vi "Teleop.vi"(10 "Match Info":T1={"Autonomous Elapsed Seconds"=0.0, "TeleOp Elapsed Seconds"=0.0, "Disabled Elapsed Seconds"=0.0, "Visited Autonomous"=FALSE, "Visited TeleOp"=FALSE, "Visited Disabled"=FALSE, "Autonomous Settings"={"Autonomous Style"=enum."Independent", "VI Refnum"=refnum}}, 11 "Call Context":T2) -> ()   [LabVIEW 2013]
doc: "This VI is called for each TeleOp packet received from the DS where the robot is not disabled. It is often used to read from the joysticks and update I/O or to update setpoints for timed control loops. It should complete and return within 20 milliseconds or it may miss DS packets."
uses:
  <vilib>/Rock Robotics/WPI/DriverStation/WPI_DriverStationDerivedRobotMode.ctl
  <vilib>/Rock Robotics/WPI/DriverStation/WPI_DriverStationMatch Info.ctl
  <vilib>/Rock Robotics/WPI/DriverStation/DriverStationLCD/WPI_DriverStationLCDLCDLine.ctl
  Begin/Robot Global Data.vi
  Begin/Global Refnums.vi
  Begin/Global Variables.vi
  <vilib>/Rock Robotics/WPI/Joystick/WPI_JoystickGetSetRefNum.vi
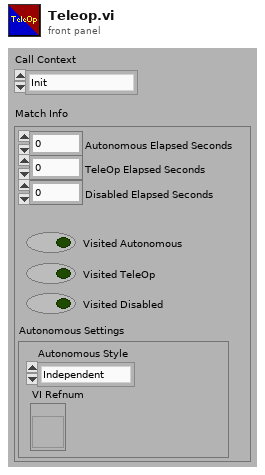
[diagram p1: front panel]
types:
  T1 = typedef "WPI_DriverStationMatch Info.ctl" = cluster{"Autonomous Elapsed Seconds":dbl, "TeleOp Elapsed Seconds":dbl, "Disabled Elapsed Seconds":dbl, "Visited Autonomous":bool, "Visited TeleOp":bool, "Visited Disabled":bool, "Autonomous Settings":cluster{"Autonomous Style":enum16{"Iterative", "Independent"}, "VI Refnum":refnum<vi>}}
  T2 = typedef "WPI_DriverStationDerivedRobotMode.ctl" = enum16{"Init", "Execute", "Stop"}
  T3 = typedef "WPI_DriverStationLCDLCDLine.ctl" = enum16{"Main - Line 1", "User - Line 2", "User - Line 3", "User - Line 4", "User - Line 5", "User - Line 6"}
  T4 = typedef "WPI_GyroDevRef.ctl" = cluster{"DevStatus":errorcluster, "Analog Module":T5, "Analog Channel":T6, "Offset":dbl, "Gain (VoltsPerDegree/Second)":dbl}
  T5 = typedef "FPGA_TypedefAnalogModule.ctl" = enum16{"Analog Module 1", "Analog Module 2"}
  T6 = typedef "FPGA_AIChannel.ctl" = enum8{"AI 1", "AI 2", "AI 3", "AI 4", "AI 5", "AI 6", "AI 7", "AI 8", "Invalid"}
  T7 = typedef "WPI_JoystickDevRef.ctl" = cluster{"Device":T8}
  T8 = typedef "WPI_JoystickDeviceEnum.ctl" = enum16{"USB 1", "USB 2", "USB 3", "USB 4", "Kinect 1", "Kinect 2"}
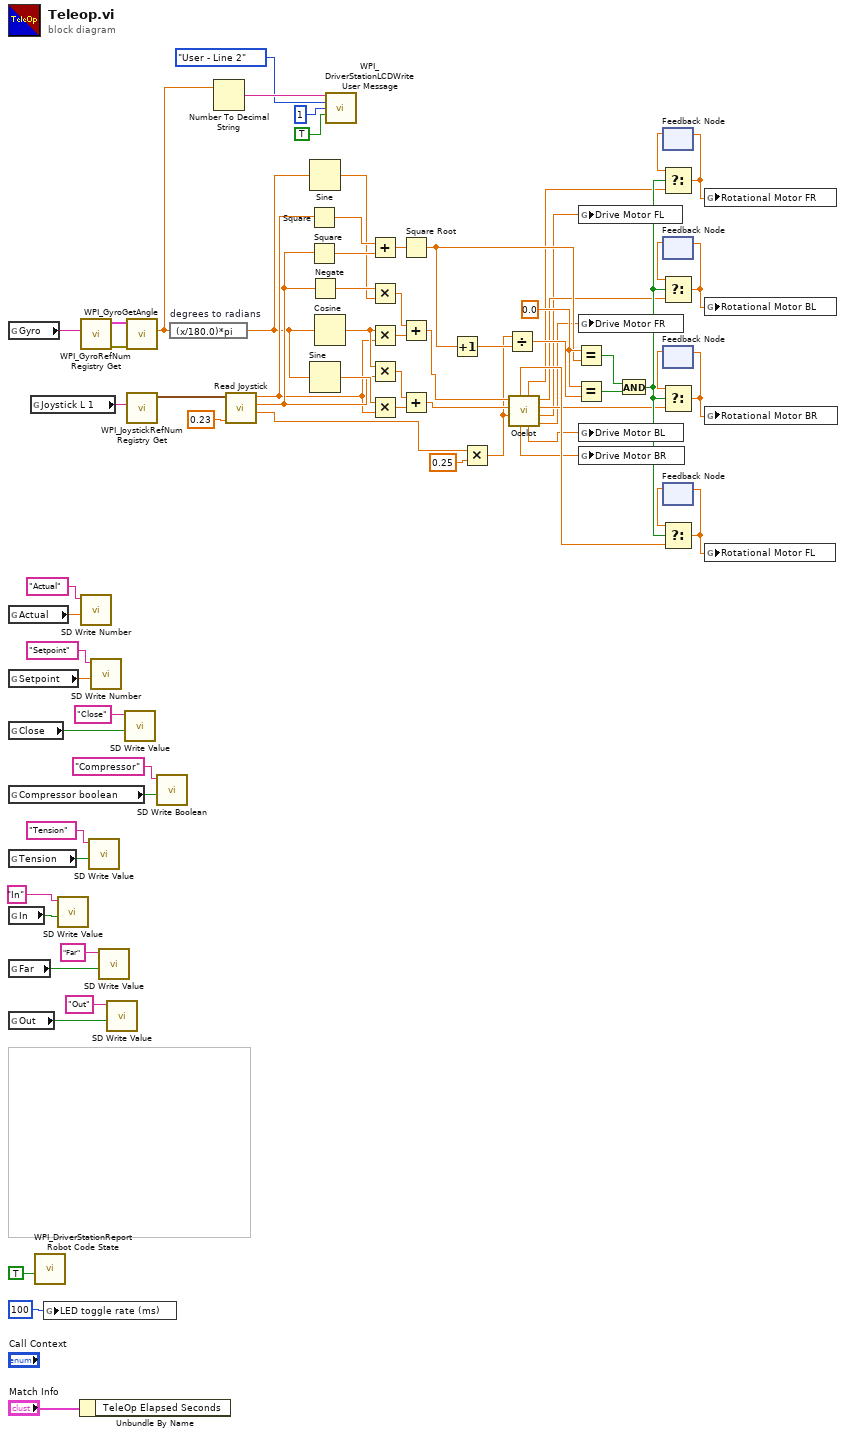
[diagram p0: block diagram]
diagram:
  w61 = 0.0 ("x")
  n1 = global read "Global Refnums.vi" "Gyro"() -> (w22:string)
  n2 = global read "Global Refnums.vi" "Actual"() -> (w37:dbl)
  n3 = global read "Global Refnums.vi" "Setpoint"() -> (w25:dbl)
  n4 = global read "Global Refnums.vi" "Close"() -> (w27:bool)
  n5 = global read "Global Refnums.vi" "Compressor boolean"() -> (w33:bool)
  n6 = global read "Global Refnums.vi" "Tension"() -> (w39:bool)
  n7 = global read "Global Refnums.vi" "In"() -> (w31:bool)
  n8 = global read "Global Refnums.vi" "Far"() -> (w35:bool)
  n9 = global read "Global Refnums.vi" "Out"() -> (w29:bool)
  n10 = global read "Global Refnums.vi" "Joystick L 1"() -> (w68:string)
  n11 = call <vilib>:"WPI_DriverStationReport Robot Code State.vi"("TeleOp"=TRUE ("Autonomous")) -> ()  [unwired: 10 in, 1 out]
  n12 = global write "Robot Global Data.vi" "LED toggle rate (ms)"(u32 100 ("LED ms toggle rate")) -> ()
  n13 = call-poly <vilib>:"SD Write Value.vi"("Boolean"=w31, "Name"="In") -> ()  [unwired: 8 in, 2 out]
  n14 = Unbundle By Name("Match Info") -> ()  [unwired: 1 out]
  n15 = call <vilib>:"WPI_GyroRefNum Registry Get.vi"("refnum name"=w22) -> ("error out"=w23:errorcluster, "GyroDevRef"=w24:T4)  [unwired: 9 in]
  n16 = call <vilib>:"SD Write Number.vi"("Numeric"=w37, "Name"="Actual") -> ()  [unwired: 8 in, 2 out]
  n17 = call-poly <vilib>:"SD Write Value.vi"("Boolean"=w39, "Name"="Tension") -> ()  [unwired: 8 in, 2 out]
  n18 = call <vilib>:"SD Write Number.vi"("Numeric"=w25, "Name"="Setpoint") -> ()  [unwired: 8 in, 2 out]
  n19 = call-poly <vilib>:"SD Write Value.vi"("Boolean"=w35, "Name"="Far") -> ()  [unwired: 8 in, 2 out]
  n20 = call-poly <vilib>:"SD Write Value.vi"("Boolean"=w29, "Name"="Out") -> ()  [unwired: 8 in, 2 out]
  n21 = call-poly <vilib>:"SD Write Value.vi"("Boolean"=w27, "Name"="Close") -> ()  [unwired: 8 in, 2 out]
  n22 = call <vilib>:"WPI_GyroGetAngle.vi"("error in (no error)"=w23, "GyroDevRef"=w24) -> ("Angle"=w5:dbl)  [unwired: 6 in, 3 out]
  n23 = call <vilib>:"WPI_JoystickRefNum Registry Get.vi"("refnum name"=w68) -> ("JoystickDevRef"=w41:T7)  [unwired: 9 in, 1 out]
  n24 = call <vilib>:"SD Write Boolean.vi"("Boolean"=w33, "Name"="Compressor") -> ()  [unwired: 8 in, 2 out]
  n25 = expression code="(x/180.0)*pi" "degrees to radians"(w5) -> (w6:dbl)
  n26 = Number To Decimal String(number=w5) -> (decimal integer string=w10:string)  [unwired: 1 in]
  n27 = call "Read Joystick.vi"("Joystick Deadbanded Value (default of 0.1)"=0.23, "Joystick L 1 DevRef"=w41) -> ("Joystick R 2 X Axis"=w2:dbl, "Joystick L 1 Y Axis"=w17:dbl, "Joystick L 1 X Axis"=w12:dbl)  [unwired: 7 in]
  n28 = Square(x=w12) -> (x^2=w66:dbl)
  n29 = Square(x=w17) -> (x^2=w67:dbl)
  n30 = Sine(x=w6) -> (sin(x)=w15:dbl)
  n31 = Negate(x=w17) -> (-x=w16:dbl)
  n32 = Sine(x=w6) -> (sin(x)=w20:dbl)
  n33 = Cosine(x=w6) -> (cos(x)=w13:dbl)
  n34 = call <vilib>:"WPI_DriverStationLCDWrite User Message.vi"("line text"=w10, "line"=WPI_DriverStationLCDLCDLine."User - Line 2", "starting column"=i8 1, "clear line before write (T)"=TRUE) -> ()  [unwired: 11 in, 1 out]
  n35 = Add(x=w66, y=w67) -> (x+y=w65:dbl)
  n36 = Multiply(x=w16, y=w15) -> (x*y=w14:dbl)
  n37 = Multiply(x=w13, y=w12) -> (x*y=w11:dbl)
  n38 = Multiply(x=w13, y=w17) -> (x*y=w21:dbl)
  n39 = Multiply(x=w20, y=w12) -> (x*y=w19:dbl)
  n40 = Square Root(x=w65) -> (sqrt(x)=w59:dbl)
  n41 = Add(x=w14, y=w11) -> (x+y=w4:dbl)
  n42 = Add(x=w21, y=w19) -> (x+y=w18:dbl)
  n43 = Increment(x=w59) -> (x+1=w60:dbl)
  n44 = Multiply(x=w2, y=0.25) -> (x*y=w1:dbl)
  n45 = Divide(x=w1, y=w60) -> (x/y=w58:dbl)
  n46 = call "Ocelot.vi"("RCW (X2)"=w1, "FWD (Y)"=w18, "STR (X)"=w4) -> ("FRD"=w52:dbl, "FLD"=w53:dbl, "BRS"=w54:dbl, "BLS"=w55:dbl, "BLD"=w51:dbl, "FRS"=w56:dbl, "BRD"=w50:dbl, "FLS"=w57:dbl)  [unwired: 1 in]
  n47 = Equal?(x=w61, y=w59) -> (x = y?=w63:bool)
  n48 = Equal?(x=w61, y=w58) -> (x = y?=w62:bool)
  n49 = global write "Global Variables.vi" "Drive Motor FL"(w53) -> ()
  n50 = global write "Global Variables.vi" "Drive Motor FR"(w52) -> ()
  n51 = global write "Global Variables.vi" "Drive Motor BL"(w51) -> ()
  n52 = global write "Global Variables.vi" "Drive Motor BR"(w50) -> ()
  n53 = And(x=w63, y=w62) -> (x .and. y?=w64:bool)
  n54 = feedback #1() -> (w48:dbl)  [unwired: 1 in]
  n55 = Select(t=w48, s=w64, f=w56) -> (s? t:f=w45:dbl)
  n56 = feedback-in #1(w45) -> ()
  n57 = feedback #2() -> (w47:dbl)  [unwired: 1 in]
  n58 = Select(t=w47, s=w64, f=w55) -> (s? t:f=w44:dbl)
  n59 = feedback-in #2(w44) -> ()
  n60 = feedback #3() -> (w46:dbl)  [unwired: 1 in]
  n61 = Select(t=w46, s=w64, f=w54) -> (s? t:f=w42:dbl)
  n62 = feedback-in #3(w42) -> ()
  n63 = feedback #4() -> (w49:dbl)  [unwired: 1 in]
  n64 = Select(t=w49, s=w64, f=w57) -> (s? t:f=w43:dbl)
  n65 = feedback-in #4(w43) -> ()
  n66 = global write "Global Variables.vi" "Rotational Motor FR"(w45) -> ()
  n67 = global write "Global Variables.vi" "Rotational Motor BL"(w44) -> ()
  n68 = global write "Global Variables.vi" "Rotational Motor BR"(w42) -> ()
  n69 = global write "Global Variables.vi" "Rotational Motor FL"(w43) -> ()
